vi "Write Data.vi"(10 "Data":i32, 11 "UPNCalculator Task Msg in":refnum<class "UPNCalculator Task Msg.lvclass">) -> (3 "UPNCalculator Task Msg out":refnum<class "UPNCalculator Task Msg.lvclass">)   [LabVIEW 2016, in "UPNCalculator Actor.lvlib" / "UPNCalculator Task Msg.lvclass"]
uses:
  UPNCalculator Task Msg.lvclass
  UPNCalculator Task Msg.lvclass/UPNCalculator Task Msg.ctl
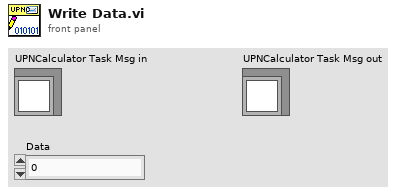
[diagram p1: front panel]
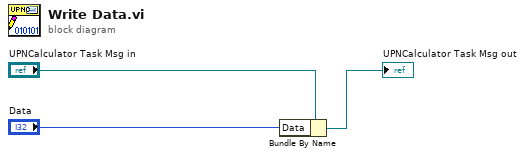
[diagram p0: block diagram]
diagram:
  n1 = Bundle By Name(cluster="UPNCalculator Task Msg in", "Data"="Data") -> (→"UPNCalculator Task Msg out":refnum<class "UPNCalculator Task Msg.lvclass">)
